vi "Encode Parameters to Words.vi"(7 "parameters":T1[](array[typedef]), 8 "error in":errorcluster, 9 "number of words":u16, 10 "values":dbl[](array[numeric]), 11 "value index":i32) -> (0 "error out":errorcluster, 3 "data words":u16[](array[numeric]) format="%04x")   [LabVIEW 2020, in "AIM MIL-STD-1553 Engine.lvlib" / "Implementation.lvlib" / "Tx Execution Unit.lvclass"]
uses:
  Tx Execution Unit.lvclass
  Tx Execution Unit.lvclass/Tx Execution Unit.ctl
  c3e650ed-1b97-4df2-943b-a2f1e3385da7.vi
  43b59857-497b-44f6-87cb-80444d0610c0.vi
  Shared/Parameter Definition.ctl
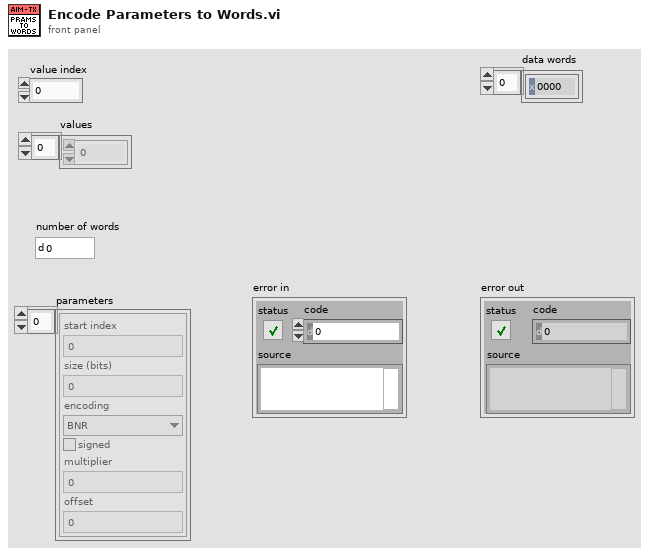
[diagram p1: front panel]
types:
  T1 = typedef "Parameter Definition.ctl" = cluster{"start index":i32, "size (bits)":i32, "encoding":enum16{"BNR", "BCD", "Discrete"}, "signed":bool, "multiplier":dbl, "offset":dbl}
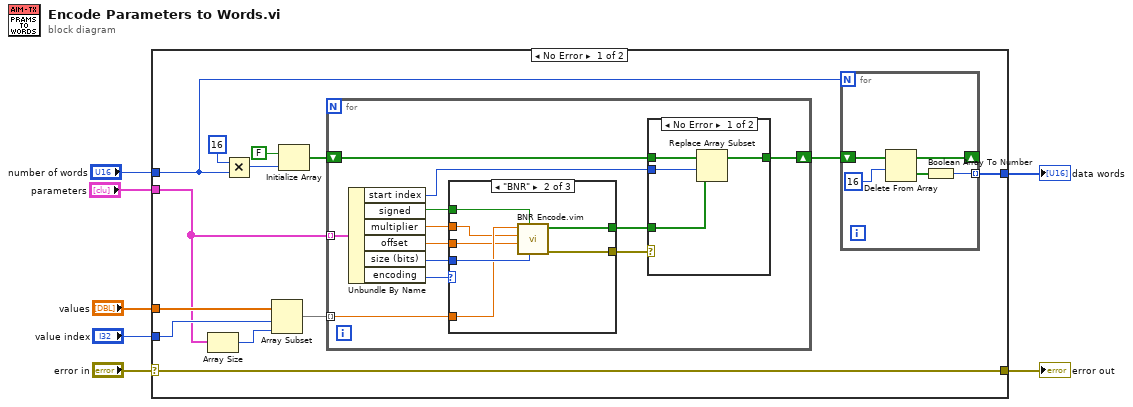
[diagram p0: block diagram]
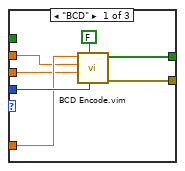
[diagram p3: hidden frame]
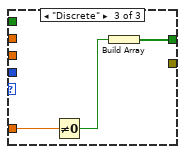
[diagram p4: hidden frame]
diagram:
  n1 = case shown="No Error" "error in" {
    selector: "error in" -> [w11 w60]
    tunnel: "parameters" -> [w9 _]
    tunnel: [w11 w60] -> w6
    tunnel: [w10 _] -> w5
    tunnel: "values" -> [w14 _]
    tunnel: "value index" -> [w13 _]
    tunnel: "number of words" -> [w8 _]
    frame No Error {
      n2 = Array Size(array=w9) -> (size(s)=w12:i32)
      n3 = Multiply(x=u16 16, y=w8) -> (x*y=w19:u16)
      n4 = Array Subset(array=w14, index=w13, length=w12) -> (w15:dbl[])
      n5 = Initialize Array(FALSE, w19) -> (w17:bool[])
      n6 = for {
        shift-right: [w27] -> w16
        shift-left: w17 -> [w28]
        tunnel: w9 -> [w37] mode=indexing
        tunnel: w15 -> [w36] mode=indexing
        n7 = Unbundle By Name(w37) -> ("start index"=w29:i32, "signed"=w34:bool, "multiplier"=w33:dbl, "offset"=w32:dbl, "size (bits)"=w31:i32, "encoding"=w35:enum16{"BNR", "BCD", "Discrete"})
        n8 = case shown="\"BNR\"" w35 {
          tunnel: w36 -> [w47 w53 w59]
          tunnel: w34 -> [_ w56 _]
          tunnel: w33 -> [w46 w52 _]
          tunnel: w32 -> [w45 w51 _]
          tunnel: w31 -> [w48 w54 _]
          tunnel: [w44 w55 _] -> w26
          tunnel: [w43 w50 w58] -> w30
          frame "BCD" {
            n9 = call "BCD Encode.vim"("data size (bits)"=w48, "signed"=FALSE, "scale offset"=w45, "scale multiplier"=w46, "value"=w47) -> ("error out"=w44:errorcluster, "BCD encoded value"=w43:bool[])  [unwired: 4 in, 1 out]
          }
          frame "BNR" {
            n10 = call "BNR Encode.vim"("data size (bits)"=w54, "signed"=w56, "scale offset"=w51, "scale multiplier"=w52, "value"=w53) -> ("error out"=w55:errorcluster, "BNR encoded value"=w50:bool[])  [unwired: 5 in]
          }
          frame "Discrete" {
            n11 = Not Equal To 0?(x=w59) -> (x != 0?=w57:bool)
            n12 = Build Array(w57) -> (w58:bool[])
          }
        }
        n13 = case shown="No Error" w26 {
          tunnel: w30 -> [w41 _]
          tunnel: w29 -> [w40 _]
          tunnel: w28 -> [w39 w42]
          tunnel: [w38 w42] -> w27
          frame No Error {
            n14 = Replace Array Subset(array=w39, new element=w41, index=w40) -> (w38:bool[])
          }
          frame Error {
            # "use previous value on error"
          }
        }
      }
      n15 = for {
        N: w8 -> [_]
        shift-right: [w24] -> _
        shift-left: w16 -> [w25]
        tunnel: [w21] -> w10 mode=indexing
        n16 = Delete From Array(array=w25, length=16 ("index")) -> (deleted portion=w22:bool[], array with subset deleted=w24:bool[])  [unwired: 1 in]
        n17 = Boolean Array To Number(Boolean array=w22) -> (number=w21:u16)
      }
    }
    frame Error {
    }
  }
  "data words" <- w5
  "error out" <- w6
